vi "PartialDischarge.vi"() -> ()   [LabVIEW 2018]
uses:
  FGV/FGV_mods.ctl
  <vilib>/Heliosphere Research LLC/Advanced Plotting Toolkit/api_core/NewPlotType.ctl
  <vilib>/Analysis/1siggen.llb/Ramp Pattern by Samples.vi
  <vilib>/Analysis/NI_AALBase.lvlib
  <vilib>/Heliosphere Research LLC/Advanced Plotting Toolkit/Advanced Plotting Toolkit.lvlib
panel:
  in  "dir_pics":path caption="Directory pictures"
  out "Progresso":dbl(slide) scale=0.0..100.0
  in  "Channels per graph":i32=1
  out "error out":errorcluster
  out "Polar":picture
  in  "file":path caption="Directory tests"
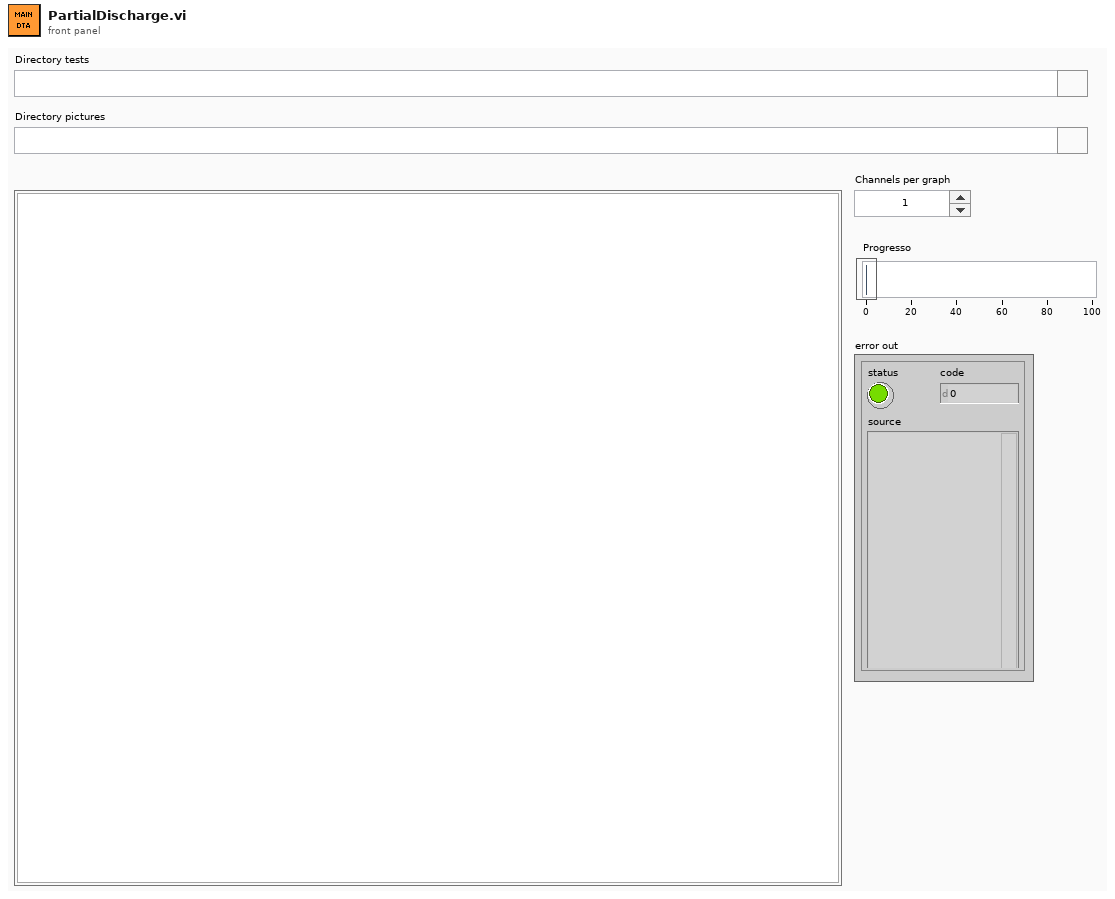
[diagram p1: front panel]
types:
  T1 = typedef "FGV_mods.ctl" = enum16{"Init", "get_config", "get_hits", "set_file", "open_file", "get_startTime", "close"}
  T2 = typedef "hit_data.ctl" = cluster{"channel":u8, "time":dbl, "parameters":cluster{"riseTime":u32, "countsToPeak":u32, "counts":u32, "energy":u32, "duration":u32, "amplitude":u32, "RMS":u32, "ASL":u32, "gain":u32, "THR":u32, "preAmp":u32, "avrFreq":u32}}
  T3 = typedef "polar_data.ctl" = cluster{"t0":dbl, "conts":dbl[], "amps":dbl[]}
  T4 = typedef "Advanced Plotting Toolkit.lvlib/NewPlotType.ctl" = enum16{"Rectangular Axes", "Polar Axes"}
  T5 = typedef "Advanced Plotting Toolkit.lvlib/PlotID.ctl" = i32
  T6 = typedef "imagedata.ctl" = cluster{"image type":i32, "image depth":i32, "image":u8[], "mask":u8[], "colors":u32[], "Rectangle":cluster{"left":i16, "top":i16, "right":i16, "bottom":i16}}
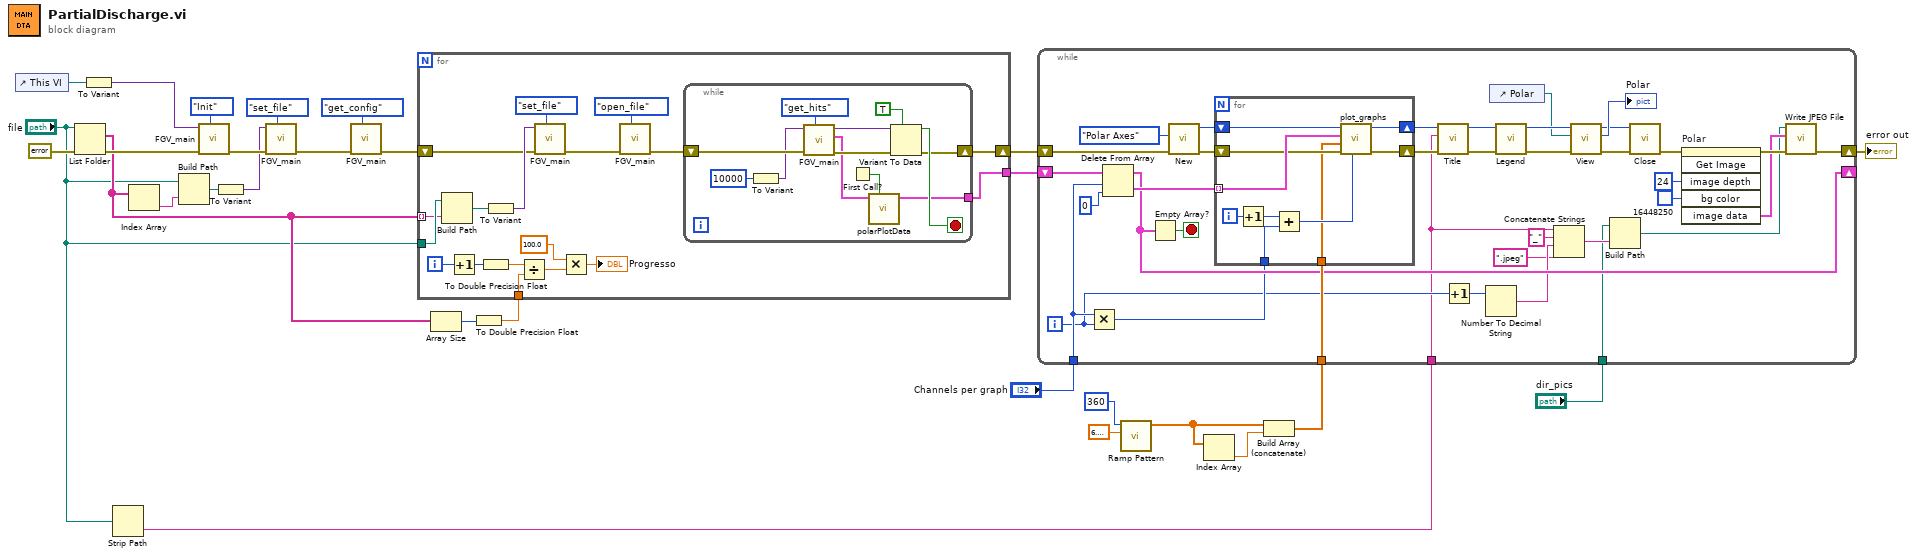
[diagram p0: block diagram]
diagram:
  n1 = control-ref of="This VI"() -> (w28:refnum<vi>)
  n2 = List Folder(path="file", error in=errorcluster {"status"=FALSE, "code"=0, "source"=""} ("Error Out")) -> (filenames=w14:string[], error out=w19:errorcluster)  [unwired: 2 in, 2 out]
  n3 = To Variant(anything=w28) -> (Variant=w20:variant)
  n4 = Strip Path(path="file") -> (name=w10:string)  [unwired: 1 out]
  n5 = Index Array(array=w14) -> (element=w25:string)  [unwired: 1 in]
  n6 = Build Path(base path="file", name or relative path=w25) -> (appended path=w24:path)
  n7 = call "FGV_main.vi"("FGV_mods"=FGV_mods."Init", "Error In"=w19, "DataIn"=w20) -> ("Error Out"=w23:errorcluster)  [unwired: 6 in, 2 out]
  n8 = To Variant(anything=w24) -> (Variant=w15:variant)
  n9 = call "FGV_main.vi"("FGV_mods"=FGV_mods."set_file", "Error In"=w23, "DataIn"=w15) -> ("Error Out"=w17:errorcluster)  [unwired: 6 in, 2 out]
  n10 = call "FGV_main.vi"("FGV_mods"=FGV_mods."get_config", "Error In"=w17) -> ("Error Out"=w16:errorcluster)  [unwired: 7 in, 2 out]
  n11 = Array Size(array=w14) -> (size(s)=w13:i32)
  n12 = To Double Precision Float(number=w13) -> (double precision float=w12:dbl)
  n13 = for {
    tunnel: [w44] -> w9
    shift-right: [w37] -> w27
    shift-left: w16 -> [w36]
    tunnel: "file" -> [w41]
    tunnel: w14 -> [w40] mode=indexing
    tunnel: w12 -> [w32]
    i -> [w35]
    n14 = Build Path(base path=w41, name or relative path=w40) -> (appended path=w39:path)
    n15 = Increment(x=w35) -> (x+1=w34:i32)
    n16 = To Double Precision Float(number=w34) -> (double precision float=w33:dbl)
    n17 = To Variant(anything=w39) -> (Variant=w38:variant)
    n18 = Divide(x=w33, y=w32) -> (x/y=w31:dbl)
    n19 = call "FGV_main.vi"("FGV_mods"=FGV_mods."set_file", "Error In"=w36, "DataIn"=w38) -> ("Error Out"=w42:errorcluster)  [unwired: 6 in, 2 out]
    n20 = Multiply(x=100.0, y=w31) -> (x*y=→"Progresso":dbl)
    n21 = call "FGV_main.vi"("FGV_mods"=FGV_mods."open_file", "Error In"=w42) -> ("Error Out"=w45:errorcluster)  [unwired: 7 in, 2 out]
    n22 = while {
      shift-right: [w51] -> w37
      shift-left: w45 -> [w57]
      tunnel: [w48] -> w44
      stop <- w52 stop-if-true
      n23 = To Variant(anything=10000) -> (Variant=w55:variant)
      n24 = call "FGV_main.vi"("FGV_mods"=FGV_mods."get_hits", "Error In"=w57, "DataIn"=w55) -> ("Error Out"=w49:errorcluster, "hits"=w47:T2[], "DataOut"=w54:variant)  [unwired: 6 in]
      n25 = First Call?() -> (First Call?: T/F=w50:bool)
      n26 = call "polarPlotData.vi"("reset"=w50, "hits"=w47) -> ("polar_plot_data"=w48:T3[])  [unwired: 9 in]
      n27 = Variant To Data(error in=w49, type=TRUE, Variant=w54) -> (data=w52:bool, error out=w51:errorcluster)
    }
  }
  n28 = call-poly <vilib>:"Ramp Pattern.vi"("end"=6.283185307179586, "samples"=360) -> ("Ramp Pattern"=w1:dbl[])  [unwired: 8 in, 1 out]
  n29 = Index Array(array=w1) -> (element=w6:dbl)  [unwired: 1 in]
  n30 = Build Array (concatenate)(w1, w6) -> (w5:dbl[])
  n31 = while {
    tunnel: w5 -> [w86]
    shift-right: [w72] -> w4
    shift-left: w27 -> [w85]
    shift-right: [w81] -> _
    shift-left: w9 -> [w84]
    tunnel: "Channels per graph" -> [w78]
    tunnel: w10 -> [w65]
    tunnel: "dir_pics" -> [w60]
    i -> [w67]
    stop <- w80 stop-if-true
    n32 = Multiply(x=w78, y=w67) -> (x*y=w79:i32)
    n33 = Delete From Array(array=w84, length=w78, index=0) -> (deleted portion=w82:T3[], array with subset deleted=w81:T3[])
    n34 = Empty Array?(array=w81) -> (empty?=w80:bool)
    n35 = call <vilib>:"New.vi"("error in (no error)"=w85, "Plot Type"=NewPlotType."Polar Axes") -> ("error out"=w92:errorcluster, "Plot ID"=w91:T5)  [unwired: 8 in]
    n36 = for {
      tunnel: w86 -> [w96]
      tunnel: w82 -> [w105] mode=indexing
      shift-right: [w102] -> w71
      shift-left: w92 -> [w104]
      shift-right: [w101] -> w68
      shift-left: w91 -> [w103]
      tunnel: w79 -> [w98]
      i -> [w100]
      n37 = Increment(x=w100) -> (x+1=w99:i32)
      n38 = Add(x=w99, y=w98) -> (x+y=w97:i32)
      n39 = call "plot_graphs.vi"("channel"=w97, "error in"=w104, "angs"=w96, "polar_data"=w105, "Plot ID"=w103) -> ("error out"=w102:errorcluster, "Plot ID out"=w101:T5)  [unwired: 5 in]
    }
    n40 = call <vilib>:"Title.vi"("error in (no error)"=w71, "Title"=w65, "Plot ID"=w68) -> ("error out"=w70:errorcluster, "Plot ID out"=w69:T5)  [unwired: 7 in]
    n41 = Increment(x=w67) -> (x+1=w66:i32)
    n42 = Number To Decimal String(number=w66) -> (decimal integer string=w64:string)  [unwired: 1 in]
    n43 = control-ref of="Polar"() -> (w90:refnum<vi>)
    n44 = call <vilib>:"Legend.vi"("error in (no error)"=w70, "Plot ID"=w69) -> ("error out"=w94:errorcluster, "Plot ID Out"=w95:T5)  [unwired: 8 in]
    n45 = Concatenate Strings(w65, "_" ("string"), w64, ".jpeg" ("string")) -> (w61:string)
    n46 = call <vilib>:"View.vi"("error in (no error)"=w94, "Ref for Sizing"=w90, "Plot ID"=w95) -> ("error out"=w88:errorcluster, "Picture"=→"Polar":picture, "Plot ID Out"=w87:T5)  [unwired: 6 in]
    n47 = Build Path(base path=w60, name or relative path=w61) -> (appended path=w59:path)
    n48 = call <vilib>:"Close.vi"("error in (no error)"=w88, "Plot ID"=w87) -> ("error out"=w77:errorcluster)  [unwired: 9 in]
    n49 = invoke on="Polar" class="Pict" method="Get Image"(error in=w77, "image depth"=24 ("Image Depth"), "bg color"=u32 16448250) -> (error out=w74:errorcluster, "image data"=w73:T6)  [unwired: 3 in, 4 out]
    n50 = call <vilib>:"Write JPEG File.vi"("error in (no error)"=w74, "image data"=w73, "path to JPEG file"=w59) -> ("error out"=w72:errorcluster)  [unwired: 7 in, 1 out]
  }
  "error out" <- w4
